vi "RDS Child Send Msg.vi"(8 "error in (no error)":errorcluster, 10 "RDS Message":refnum<class "RDS Message.lvclass">, 11 "RDS Parent Actor in":refnum<class "RDS Parent Actor.lvclass">) -> (0 "error out":errorcluster, 3 "RDS Parent Actor out":refnum<class "RDS Parent Actor.lvclass">)   [LabVIEW 2015, in "RDS Abstracts.lvlib" / "RDS Parent Actor.lvlib" / "RDS Parent Actor.lvclass"]
uses:
  RDS Parent Actor.lvclass
  Libraries/RDS Framework/RDS Message Class/RDS Message.lvclass
  RDS Parent Actor.lvclass/RDS Parent Actor.ctl
  RDS Router Actor/RDS Router Actor Messages/RSD Msg Send To Router Msg/RSD Msg Send To Router Msg.lvclass
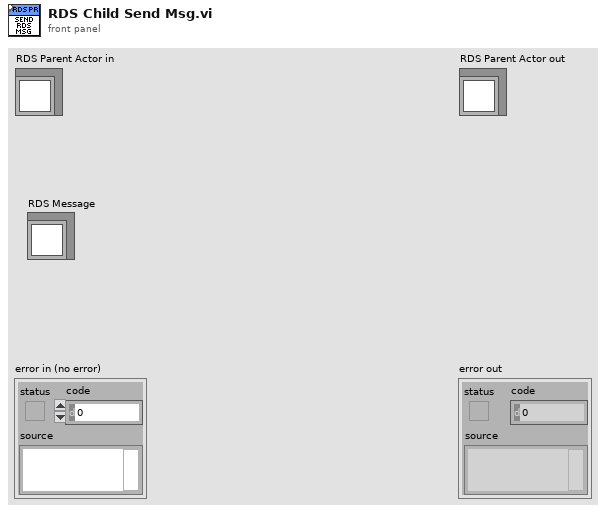
[diagram p1: front panel]
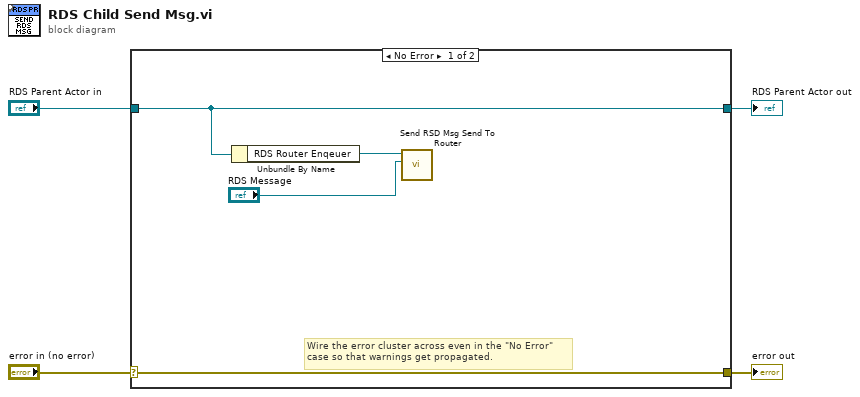
[diagram p0: block diagram]
diagram:
  n1 = case shown="No Error" "error in (no error)" {
    selector: "error in (no error)" -> [w8 w10]
    tunnel: [w8 w10] -> w3
    tunnel: [w7 w9] -> w1
    tunnel: "RDS Parent Actor in" -> [w7 w9]
    frame No Error {
      # "Wire the error cluster across even in the \"No Error\"\ncase so that warnings get propagated."
      n2 = Unbundle By Name(w7) -> ("RDS Router Enqeuer"=w6:refnum<class "Message Enqueuer.lvclass">)
      n3 = call "Send RSD Msg Send To Router.vi"("RDS Message"="RDS Message", "Message Enqueuer in"=w6) -> ()  [unwired: 8 in, 2 out]
    }
    frame Error {
    }
  }
  "error out" <- w3
  "RDS Parent Actor out" <- w1
